vi "Store Configuration List.vi"(0 "VISA resource name":refnum<visa-resource-name>, 1 "Configuration List Type (0: Measure)":u16(ring) items=["Measure", "Source"], 2 "Configuration List Name":string="myList", 3 "Specify Configuration Point (T:Yes)":bool=TRUE, 4 "Configuration Point index (1)":u32=1 min=1, 5 "error in (no error)":errorcluster) -> (14 "VISA resource name out":refnum<visa-resource-name>, 19 "error out":errorcluster)   [LabVIEW 2018, in "Keithley 2450.lvlib"]
doc: "Stores the active instrument settings into the named Measure or Source Configuration List."
uses:
  <instrlib>/Keithley 2450/Keithley 2450.lvlib
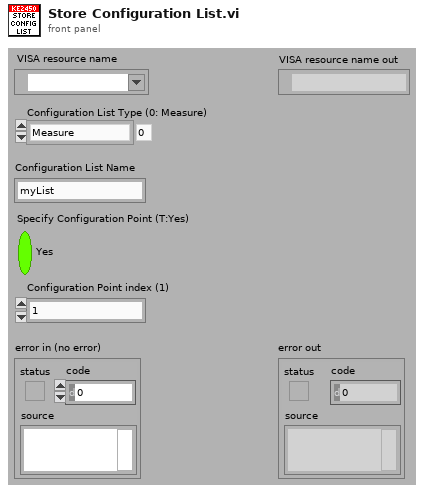
[diagram p1: front panel]
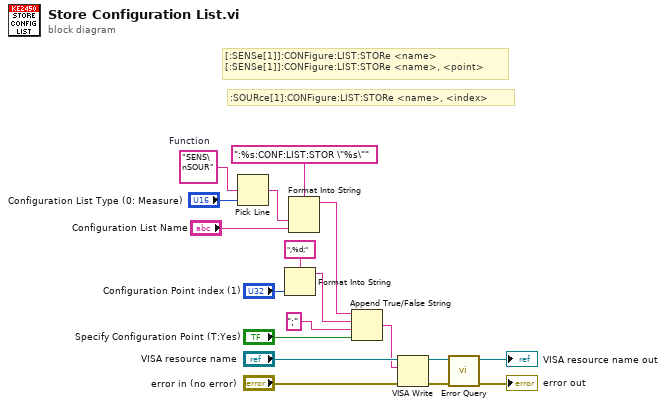
[diagram p0: block diagram]
diagram:
  w14 = "SENS\nSOUR"  # Function
  # "[:SENSe[1]]:CONFigure:LIST:STORe <name>\n[:SENSe[1]]:CONFigure:LIST:STORe <name>, <point>"
  # ":SOURce[1]:CONFigure:LIST:STORe <name>, <index>"
  n1 = Pick Line(multi-line string=w14, line index="Configuration List Type (0: Measure)") -> (output string=w9:string)  [unwired: 1 out]
  n2 = Format Into String(format string=",%d;", "Configuration Point index (1)") -> (resulting string=w4:string)  [unwired: 2 in, 1 out]
  n3 = Format Into String(format string=":%s:CONF:LIST:STOR \"%s\"", w9, "Configuration List Name") -> (resulting string=w2:string)  [unwired: 2 in, 1 out]
  n4 = Append True/False String(1:"Specify Configuration Point (T:Yes)", 2:";" ("false string"), 3:w4, 4:w2) -> (0:w1:string)
  n5 = VISA Write(VISA resource name="VISA resource name", write buffer=w1, error in (no error)="error in (no error)") -> (VISA resource name out=w12:refnum<visa-resource-name>, error out=w11:errorcluster)  [unwired: 1 out]
  n6 = call <instrlib>:"Error Query.vi"("error in (no error)"=w11, "VISA resource name"=w12) -> ("error out"=→"error out":errorcluster, "VISA resource name out"=→"VISA resource name out":refnum<visa-resource-name>)  [unwired: 8 out]
